vi "WPI_DashboardProcessStatusPacket.vi"(11 "data in":string) -> (1 "Disconnected":bool, 2 "Robot Metrics":T1, 3 "Status Cluster":T2)   [LabVIEW 2025]
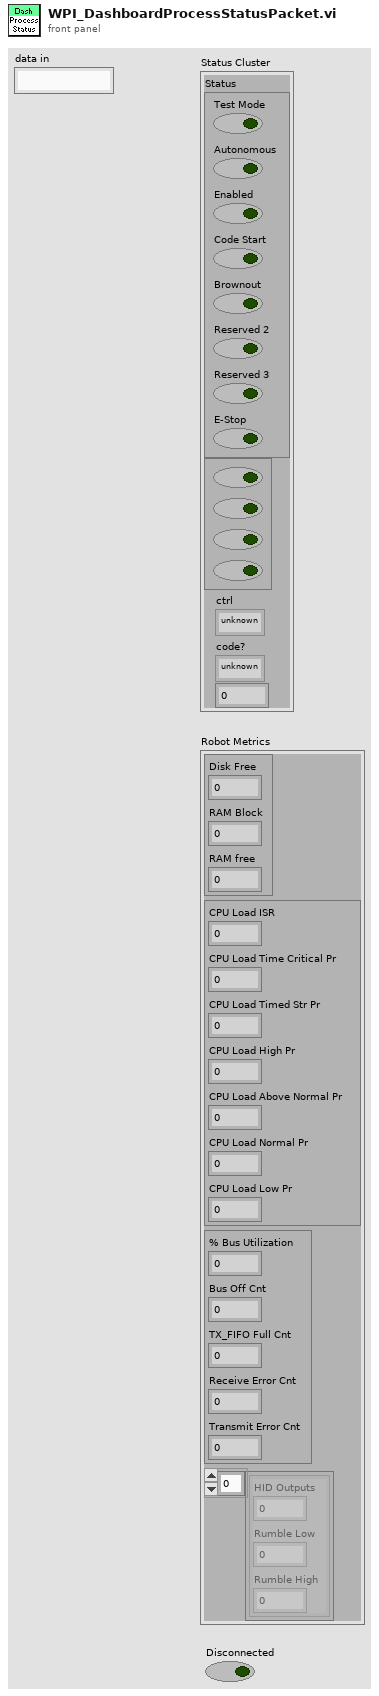
[diagram p1: front panel]
types:
  T1 = cluster{cluster{"Disk Free":u64, "RAM Block":u32, "RAM free":u32}, cluster{"CPU Load ISR":sgl, "CPU Load Time Critical Pr":sgl, "CPU Load Timed Str Pr":sgl, "CPU Load High Pr":sgl, "CPU Load Above Normal Pr":sgl, "CPU Load Normal Pr":sgl, "CPU Load Low Pr":sgl}, cluster{"% Bus Utilization":sgl, "Bus Off Cnt":u32, "TX_FIFO Full Cnt":u32, "Receive Error Cnt":u8, "Transmit Error Cnt":u8}, cluster{"HID Outputs":u32, "Rumble Low":u16, "Rumble High":u16}[]}
  T2 = cluster{"Status":cluster{"Test Mode":bool, "Autonomous":bool, "Enabled":bool, "Code Start":bool, "Brownout":bool, "Reserved 2":bool, "Reserved 3":bool, "E-Stop":bool}, cluster{bool, bool, bool, bool}, "ctrl":enum16{"unknown", "cRIO", "roboRio"}, "code?":enum16{"unknown", "noCode", "code"}, dbl}
  T3 = cluster{"Packet Number":u16, "Version":u8, "Status":u8, "Trace":u8, "Battery":cluster{"Int":u8, "Dec":u8}}
  T4 = cluster{"Disk Free":u64, "RAM Block":u32, "RAM free":u32, cluster{"CPU Load ISR":sgl, "CPU Load Time Critical Pr":sgl, "CPU Load Timed Str Pr":sgl, "CPU Load High Pr":sgl, "CPU Load Above Normal Pr":sgl, "CPU Load Normal Pr":sgl, "CPU Load Low Pr":sgl}, cluster{"% Bus Utilization":sgl, "Bus Off Cnt":u32, "TX_FIFO Full Cnt":u32, "Receive Error Cnt":u8, "Transmit Error Cnt":u8}, cluster{"HID Outputs":u32, "Rumble Low":u16, "Rumble High":u16}[]}
  T5 = cluster{"Packet Number":u16, "Version":u8, "Status":u8, "Trace":u8, "Battery":cluster{"Int":u8, "Dec":u8}, "Request":u8}
  T6 = cluster{"Test Mode":bool, "Autonomous":bool, "Enabled":bool, "Code Start":bool, "Brownout":bool, "Reserved 2":bool, "Reserved 3":bool, "E-Stop":bool}
  T7 = cluster{"HID Outputs":u32, "Rumble Low":u16, "Rumble High":u16}
  T8 = cluster{"CPU Low":sgl, "CPU Normal":sgl, "CPU TC":sgl, "CPU Int":sgl}
  T9 = cluster{"% Bus Utilization":sgl, "Bus Off Cnt":u32, "TX_FIFO Full Cnt":u32, "Receive Error Cnt":u8, "Transmit Error Cnt":u8}
  T10 = cluster{"HID Outputs":u32, "Rumble Low":u16, "Rumble High":u16}[]
  T11 = cluster{"CPU Load ISR":sgl, "CPU Low":sgl, "CPU Load ISR":sgl, "CPU Load ISR":sgl, "CPU Normal":sgl, "CPU TC":sgl, "CPU Int":sgl}
  T12 = cluster{"CPU Load ISR":sgl, "CPU Load Time Critical Pr":sgl, "CPU Load Timed Str Pr":sgl, "CPU Load High Pr":sgl, "CPU Load Above Normal Pr":sgl, "CPU Load Normal Pr":sgl, "CPU Load Low Pr":sgl}
  T13 = cluster{"Disk Free":u64, "RAM Block":u32, "RAM free":u32}
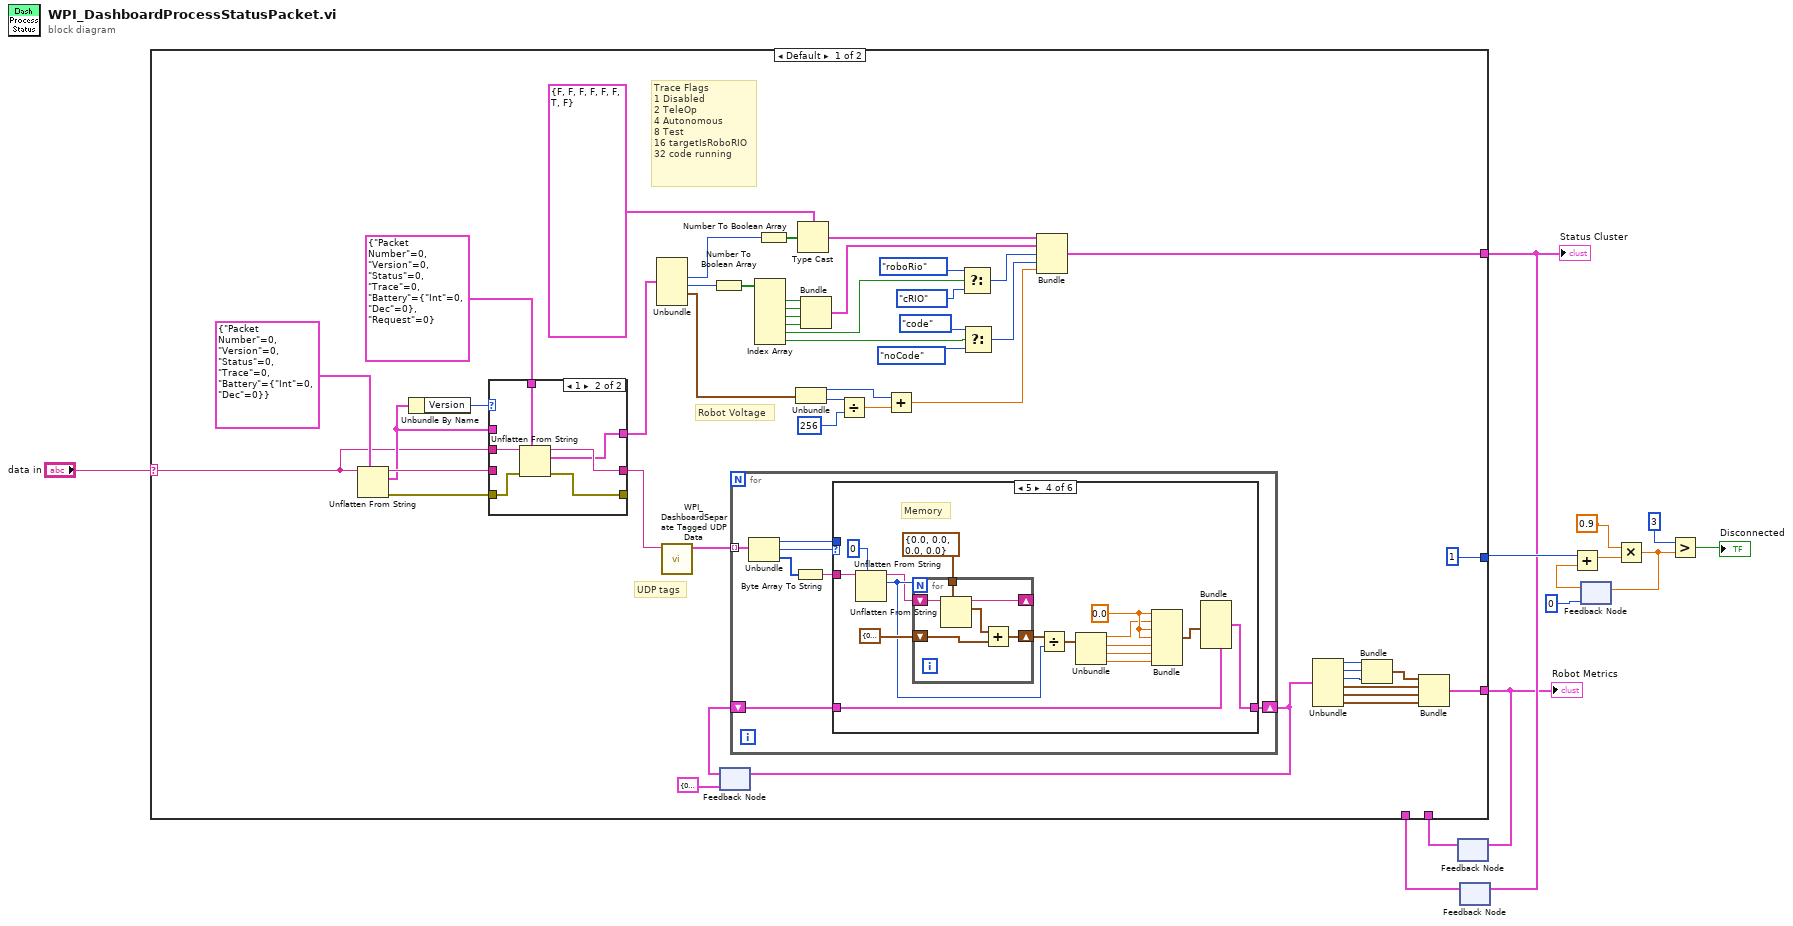
[diagram p0: block diagram]
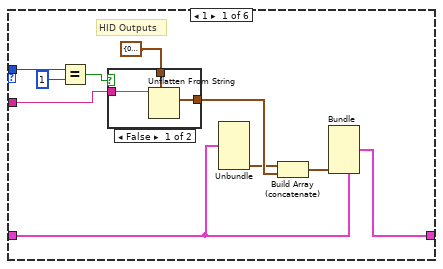
[diagram p2: hidden frame]
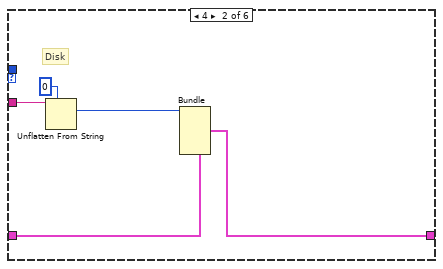
[diagram p4: hidden frame]
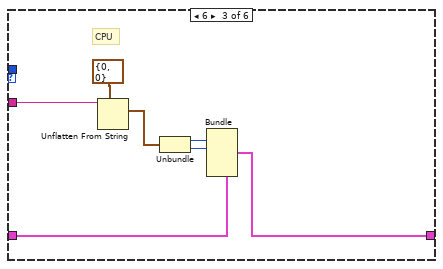
[diagram p5: hidden frame]
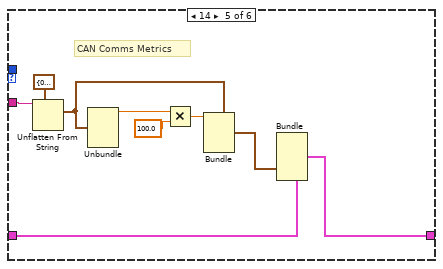
[diagram p6: hidden frame]
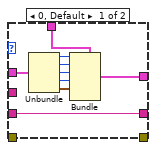
[diagram p8: hidden frame]
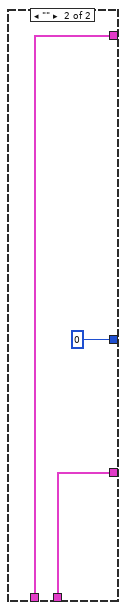
[diagram p9: hidden frame]
diagram:
  n1 = feedback #1() -> (w3:T1)  [unwired: 1 in]
  n2 = feedback #2() -> (w4:T2)  [unwired: 1 in]
  n3 = case shown="Default" "data in" {
    selector: "data in" -> [w14 _]
    tunnel: [w17 w142] -> w2
    tunnel: [w16 w143] -> w5
    tunnel: w3 -> [_ w142]
    tunnel: w4 -> [_ w143]
    tunnel: [1 0] -> w6
    frame Default {
      # "UDP tags"
      # "Trace Flags\n1 Disabled\n2 TeleOp\n4 Autonomous\n8 Test\n16 targetIsRoboRIO\n32 code running"
      # "Robot Voltage"
      n4 = Unflatten From String(type=T3 {"Packet Number"=0, "Version"=0, "Status"=0, "Trace"=0, "Battery"={"Int"=0, "Dec"=0}}, binary string=w14) -> (rest of the binary string=w57:string, value=w56:T3, error out=w51:errorcluster)  [unwired: 1 in, 2 out]
      n5 = Unbundle By Name(w56) -> ("Version"=w58:u8)
      n6 = case shown="1" w58 {
        tunnel: w56 -> [w134 _]
        tunnel: w57 -> [w126 _]
        tunnel: [w127 w137] -> w55
        tunnel: T5 {"Packet Number"=0, "Version"=0, "Status"=0, "Trace"=0, "Battery"={"Int"=0, "Dec"=0}, "Request"=0} -> [w133 w140]
        tunnel: [w126 w138] -> w52
        tunnel: w14 -> [_ w139]
        tunnel: w51 -> [_ w136]
        tunnel: [_ w135] -> _
        frame 0, Default {
          n7 = Unbundle(w134) -> ("Packet Number"=w132:u16, "Version"=w131:u8, "Status"=w130:u8, "Trace"=w129:u8, "Battery"=w128:cluster{"Int":u8, "Dec":u8})
          n8 = Bundle(cluster=w133, "Packet Number"=w132, "Version"=w131, "Status"=w130, "Trace"=w129, "Battery"=w128) -> (w127:T5)  [unwired: 1 in]
        }
        frame 1 {
          n9 = Unflatten From String(type=w140, binary string=w139, error in (no error)=w136) -> (rest of the binary string=w138:string, value=w137:T5, error out=w135:errorcluster)  [unwired: 2 out]
        }
      }
      n10 = Unbundle(w55) -> ("Status"=w60:u8, "Trace"=w38:u8, "Battery"=w40:cluster{"Int":u8, "Dec":u8})  [unwired: 3 out]
      n11 = call <vilib>:"WPI_DashboardSeparate Tagged UDP Data.vi"("String"=w52) -> ("Tagged Array"=w26:cluster{u8, u8, "unsigned byte array":u8[]}[])  [unwired: 10 in]
      n12 = Number To Boolean Array(number=w38) -> (Boolean array=w37:bool[])
      n13 = feedback #3(T4 {"Disk Free"=0, "RAM Block"=0, "RAM free"=0, {"CPU Load ISR"=0.0, "CPU Load Time Critical Pr"=0.0, "CPU Load Timed Str Pr"=0.0, "CPU Load High Pr"=0.0, "CPU Load Above Normal Pr"=0.0, "CPU Load Normal Pr"=0.0, "CPU Load Low Pr"=0.0}, {"% Bus Utilization"=0.0, "Bus Off Cnt"=0, "TX_FIFO Full Cnt"=0, "Receive Error Cnt"=0, "Transmit Error Cnt"=0}, []} ("Profile Data")) -> (w27:T4)
      n14 = for {
        tunnel: w26 -> [w68] mode=indexing
        shift-right: [w65] -> w25
        shift-left: w27 -> [w66]
        n15 = Unbundle(w68) -> (w62:u8, w67:u8, "unsigned byte array"=w64:u8[])
        n16 = Byte Array To String(unsigned byte array=w64) -> (string=w63:string)
        n17 = case shown="5" w67 {
          tunnel: w66 -> [w72 w86 w93 w109 w118 w125]
          tunnel: [w78 w85 w92 w108 w117 w125] -> w65
          tunnel: w63 -> [w74 w84 w91 w107 w119 _]
          tunnel: w62 -> [w75 _ _ _ _ _]
          frame 1 {
            # "HID Outputs"
            n18 = Equal?(x=w75, y=u8 1) -> (x = y?=w77:bool)
            n19 = case shown="False" w77 {
              tunnel: w74 -> [w81 _]
              tunnel: T7 {"HID Outputs"=0, "Rumble Low"=0, "Rumble High"=0} -> [w80 _]
              tunnel: [w79 _] -> w71
              frame False {
                n20 = Unflatten From String(type=w80, binary string=w81) -> (value=w79:T7)  [unwired: 3 in, 2 out]
              }
              frame True {
              }
            }
            n21 = Unbundle(w72) -> (w69:T10)  [unwired: 5 out]
            n22 = Build Array (concatenate)(w69, w71) -> (w70:T10)
            n23 = Bundle(cluster=w72, w70) -> (w78:T4)  [unwired: 5 in]
          }
          frame 4 {
            # "Disk"
            n24 = Unflatten From String(type=u64 0 ("Disk Free"), binary string=w84) -> (value=w82:u64)  [unwired: 3 in, 2 out]
            n25 = Bundle(cluster=w86, "Disk Free"=w82) -> (w85:T4)  [unwired: 5 in]
          }
          frame 6 {
            # "CPU"
            n26 = Unflatten From String(type=cluster{"Disk Free":u32, "Disk Free 2":u32} {"Disk Free"=0, "Disk Free 2"=0}, binary string=w91) -> (value=w89:cluster{"Disk Free":u32, "Disk Free 2":u32})  [unwired: 3 in, 2 out]
            n27 = Unbundle(w89) -> ("Disk Free"=w88:u32, "Disk Free 2"=w87:u32)
            n28 = Bundle(cluster=w93, "RAM Block"=w88, "RAM free"=w87) -> (w92:T4)  [unwired: 4 in]
          }
          frame 5 {
            w99 = sgl 0.0 ("CPU Load ISR")
            # "Memory"
            n29 = Unflatten From String(type=u8 0, binary string=w107) -> (rest of the binary string=w100:string, value=w103:u8)  [unwired: 3 in, 1 out]
            n30 = for {
              N: w103 -> [_]
              tunnel: T8 {"CPU Low"=0.0, "CPU Normal"=0.0, "CPU TC"=0.0, "CPU Int"=0.0} -> [w115]
              shift-right: [w112] -> w102
              shift-left: T8 {"CPU Low"=0.0, "CPU Normal"=0.0, "CPU TC"=0.0, "CPU Int"=0.0} -> [w114]
              shift-right: [w110] -> _
              shift-left: w100 -> [w111]
              n31 = Unflatten From String(type=w115, binary string=w111) -> (rest of the binary string=w110:string, value=w113:T8)  [unwired: 3 in, 1 out]
              n32 = Add(x=w113, y=w114) -> (x+y=w112:T8)
            }
            n33 = Divide(x=w102, y=w103) -> (x/y=w101:T8)
            n34 = Unbundle(w101) -> ("CPU Low"=w94:sgl, "CPU Normal"=w95:sgl, "CPU TC"=w96:sgl, "CPU Int"=w97:sgl)
            n35 = Bundle("CPU Load ISR"=w99, "CPU Low"=w94, "CPU Load ISR"=w99, "CPU Load ISR"=w99, "CPU Normal"=w95, "CPU TC"=w96, "CPU Int"=w97) -> (w98:T11)  [unwired: 1 in]
            n36 = Bundle(cluster=w109, w98) -> (w108:T4)  [unwired: 5 in]
          }
          frame 14 {
            # "CAN Comms Metrics"
            n37 = Unflatten From String(type=T9 {"% Bus Utilization"=0.0, "Bus Off Cnt"=0, "TX_FIFO Full Cnt"=0, "Receive Error Cnt"=0, "Transmit Error Cnt"=0}, binary string=w119) -> (value=w121:T9)  [unwired: 3 in, 2 out]
            n38 = Unbundle(w121) -> ("% Bus Utilization"=w122:sgl)  [unwired: 4 out]
            n39 = Multiply(x=w122, y=sgl 100.0) -> (x*y=w123:sgl)
            n40 = Bundle(cluster=w121, "% Bus Utilization"=w123) -> (w116:T9)  [unwired: 4 in]
            n41 = Bundle(cluster=w118, w116) -> (w117:T4)  [unwired: 5 in]
          }
          frame Default {
          }
        }
      }
      n42 = feedback-in #3(w25) -> ()
      n43 = Index Array(array=w37) -> (element #1=w36:bool, element #2=w35:bool, element #3=w34:bool, element #4=w33:bool, element #5=w32:bool, element #6=w31:bool)  [unwired: 6 in]
      n44 = Number To Boolean Array(number=w60) -> (Boolean array=w61:bool[])
      n45 = Unbundle(w40) -> ("Int"=w41:u8, "Dec"=w44:u8)
      n46 = Type Cast(type=T6 {"Test Mode"=FALSE, "Autonomous"=FALSE, "Enabled"=FALSE, "Code Start"=FALSE, "Brownout"=FALSE, "Reserved 2"=FALSE, "Reserved 3"=TRUE, "E-Stop"=FALSE} ("Status"), x=w61) -> (*(type *) &x=w29:T6)
      n47 = Bundle(w36, w35, w34, w33) -> (w30:cluster{bool, bool, bool, bool})  [unwired: 1 in]
      n48 = Divide(x=w44, y=256) -> (x/y=w42:dbl)
      n49 = Add(x=w41, y=w42) -> (x+y=w39:dbl)
      n50 = Select(t=enum16{"unknown", "cRIO", "roboRio"}."roboRio" ("ctrl"), s=w32, f=enum16{"unknown", "cRIO", "roboRio"}."cRIO" ("ctrl")) -> (s? t:f=w48:enum16{"unknown", "cRIO", "roboRio"})
      n51 = Select(t=enum16{"unknown", "noCode", "code"}."code" ("code?"), s=w31, f=enum16{"unknown", "noCode", "code"}."noCode" ("code?")) -> (s? t:f=w45:enum16{"unknown", "noCode", "code"})
      n52 = Bundle("Status"=w29, w30, "ctrl"=w48, "code?"=w45, w39) -> (w16:T2)  [unwired: 1 in]
      n53 = Unbundle(w25) -> ("Disk Free"=w24:u64, "RAM Block"=w23:u32, "RAM free"=w22:u32, w20:T12, w19:T9, w18:T10)
      n54 = Bundle("Disk Free"=w24, "RAM Block"=w23, "RAM free"=w22) -> (w21:T13)  [unwired: 1 in]
      n55 = Bundle(w21, w20, w19, w18) -> (w17:T1)  [unwired: 1 in]
    }
    frame "" {
    }
  }
  "Status Cluster" <- w5
  "Robot Metrics" <- w2
  n56 = feedback-in #1(w2) -> ()
  n57 = feedback-in #2(w5) -> ()
  n58 = feedback #4(0) -> (w7:dbl)
  n59 = Add(x=w6, y=w7) -> (x+y=w8:dbl)
  n60 = Multiply(x=0.9, y=w8) -> (x*y=w11:dbl)
  n61 = feedback-in #4(w11) -> ()
  n62 = Greater?(x=3, y=w11) -> (0:→"Disconnected":bool)
